vi "InitWrist V2.vi"() -> ()   [LabVIEW 2015]
uses:
  <vilib>/myRIO/Common/Instrument Driver Framework/myRIO v1.0/Encoder/typedefs/Encoder Signal Mode.ctl
  <vilib>/myRIO/Instrument Drivers/Onboard IO/Encoder/typedefs/Encoder Reference.ctl
  <vilib>/myRIO/Common/Instrument Driver Framework/Utilities/typedefs/myRIO Generic Hardware Reference.ctl
  <vilib>/myRIO/Common/Instrument Driver Framework/Utilities/typedefs/Hardware Version Enum.ctl
  <vilib>/myRIO/Common/Instrument Driver Framework/Utilities/typedefs/myRIO v1.0 Reference.ctl
  <vilib>/myRIO/Common/Instrument Driver Framework/Utilities/typedefs/Generic FPGA Reference.ctl
  <vilib>/myRIO/Common/Instrument Driver Framework/myRIO v1.0/Encoder/typedefs/Encoder Channels Enum.ctl
  <vilib>/myRIO/Common/Instrument Driver Framework/myRIO v1.0/Encoder/typedefs/Encoder Configuration v1.0.ctl
  <vilib>/userdefined/High Color/nirio_resource_hc.ctl
  <vilib>/myRIO/Instrument Drivers/Onboard IO/DIO/typedefs/DIO Reference.ctl
  <vilib>/myRIO/Common/Instrument Driver Framework/myRIO v1.0/DIO/typedefs/DIO Channels List.ctl
  <vilib>/myRIO/Common/Instrument Driver Framework/myRIO v1.0/DIO/typedefs/DIO Channels Enum.ctl
  <vilib>/myRIO/Common/Instrument Driver Framework/Utilities/vis/Is FPGA Ref Available.vi
  <vilib>/myRIO/Common/Instrument Driver Framework/myRIO v1.0/Encoder/vis/myRIO v1.1 Open Encoder.vi
  <vilib>/myRIO/Instrument Drivers/Onboard IO/Encoder/vis/Read.vi
  <vilib>/myRIO/Common/Instrument Driver Framework/myRIO v1.0/DIO/vis/myRIO v1.1 Open DIO.vi
  <vilib>/myRIO/Instrument Drivers/Onboard IO/DIO/vis/Read.vi
  <vilib>/myRIO/Common/Instrument Driver Framework/Utilities/vis/Validate Channels.vi
  <vilib>/myRIO/Common/Instrument Driver Framework/myRIO v1.0/Encoder/vis/myRIO v1.0 Reserve Encoder.vi
  <vilib>/myRIO/Common/Instrument Driver Framework/myRIO v1.0/DIO/vis/myRIO v1.0 Reserve DIO.vi
  <vilib>/myRIO/Common/Instrument Driver Framework/myRIO v1.0/Encoder/vis/myRIO v1.0 Build MUX Configuration Encoder.vi
  <vilib>/myRIO/Common/Instrument Driver Framework/myRIO v1.0/Resource Manager/vis/myRIO v1.0 Reserve Channel List.vi
  <vilib>/myRIO/Common/Instrument Driver Framework/myRIO v1.0/DIO/vis/myRIO v1.0 Build MUX Configuration DIO.vi
  <vilib>/myRIO/Common/Instrument Driver Framework/myRIO v1.0/Resource Manager/vis/myRIO v1.0 Create Configuration List.vi
  <vilib>/myRIO/Common/Instrument Driver Framework/myRIO v1.0/Resource Manager/vis/myRIO v1.0 Reserve Channel.vi
  <vilib>/myRIO/Common/Instrument Driver Framework/myRIO v1.0/Resource Manager/vis/myRIO v1.0 Unreserve Channel.vi
  <vilib>/myRIO/Common/Instrument Driver Framework/myRIO v1.0/Resource Manager/vis/myRIO v1.0 Build Mutex Name.vi
  Global Angle.vi
  <vilib>/Utility/VariantDataType/GetNumericInfo.vi
  <vilib>/Utility/error.llb/Error Cluster From Error Code.vi
  <vilib>/myRIO/Common/Instrument Driver Framework/myRIO v1.0/myRIO v1.1 Open.vi
  <vilib>/myRIO/Common/Instrument Driver Framework/Utilities/vis/IO Manager.vi
  <vilib>/myRIO/Common/Instrument Driver Framework/Utilities/vis/Configuration Manager.vi
  <vilib>/myRIO/Common/Instrument Driver Framework/myRIO v1.0/Resource Manager/vis/myRIO v1.0 Configure IO.vi
  <vilib>/myRIO/Common/Instrument Driver Framework/myRIO v1.0/myRIO v1.0 Close.vi
  <vilib>/myRIO/Common/Instrument Driver Framework/myRIO v1.0/Encoder/vis/myRIO v1.0 Configure Encoder.vi
  <vilib>/myRIO/Common/Instrument Driver Framework/myRIO v1.0/Encoder/vis/myRIO v1.0 Read Encoder.vi
  <vilib>/myRIO/Common/Instrument Driver Framework/myRIO v1.0/DIO/vis/myRIO v1.0 Read DIO.vi
  <vilib>/myRIO/Express VI/Onboard IO/Encoder/Encoder Express VI.xnode
  <vilib>/myRIO/Instrument Drivers/Onboard IO/Encoder/vis/myRIO Encoder Open.xnode
  <vilib>/myRIO/Common/Instrument Driver Framework/myRIO v1.0/Encoder/typedefs/Encoder Count Direction Enum.ctl
  <vilib>/myRIO/Express VI/Onboard IO/DI/DI Express VI.xnode
  <vilib>/myRIO/Instrument Drivers/Onboard IO/DIO/vis/myRIO DIO Open.xnode
  <vilib>/myRIO/Instrument Drivers/Onboard IO/Encoder/Encoder.lvlib
  <vilib>/myRIO/Instrument Drivers/Onboard IO/DIO/DIO.lvlib
panel:
  out ".not. x?":bool
  in  "integral":dbl
  out "Boolean":bool
  out "lastError":dbl
  in  "stop":bool
  out "Counter Value":i32
  out "input Rotations":dbl
  out "error":i32
  out "motorStop":bool
  out "differential":i32
  out "output":i32
  out "busy":bool
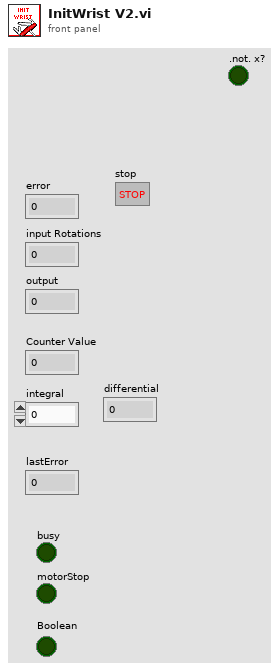
[diagram p1: front panel]
types:
  T1 = typedef "Encoder.lvlib/Encoder Reference.ctl" = cluster{"myRIO Reference":T2, "Encoder Channels Enum":T6}
  T2 = typedef "myRIO Generic Hardware Reference.ctl" = cluster{"myRIO Model":T3, "myRIO Hardware Reference":T4}
  T3 = typedef "Hardware Version Enum.ctl" = enum16{"Unknown", "myRIO-1900", "myRIO-1950", "roboRIO"}
  T4 = typedef "myRIO v1.0 Reference.ctl" = cluster{"Generic FPGA Reference":T5, "Allow multiple opens":bool}
  T5 = typedef "Generic FPGA Reference.ctl" = refnum<k20>
  T6 = typedef "Encoder Channels Enum.ctl" = enum16{"Not Connected", "C/ENC0", "C/ENC1", "A/ENC", "B/ENC", "DIO/ENC0", "DIO/ENC1", "DIO/ENC2", "DIO/ENC3", "DIO/ENC4"}
  T7 = typedef "Encoder Signal Mode.ctl" = enum16{"Quadrature phase signal", "Step and direction signal"}
  T8 = typedef "nirio_resource_hc.ctl" = tag
  T9 = typedef "DIO.lvlib/DIO Reference.ctl" = cluster{"myRIO Reference":T2, "DIO Channels List":T10}
  T10 = typedef "DIO Channels List.ctl" = T11[]
  T11 = typedef "DIO Channels Enum.ctl" = enum16{"Not Connected", "C/DIO0", "C/DIO1", "C/DIO2", "C/DIO3", "C/DIO4", "C/DIO5", "C/DIO6", "C/DIO7", "A/DIO0", "A/DIO1", "A/DIO2", "A/DIO3", "A/DIO4", "A/DIO5", "A/DIO6", "A/DIO7", "A/DIO8", "A/DIO9", "A/DIO10", "A/DIO11", "A/DIO12", "A/DIO13", "A/DIO14", "A/DIO15", "B/DIO0", "B/DIO1", "B/DIO2", "B/DIO3", "B/DIO4", "B/DIO5", "B/DIO6", "B/DIO7", "B/DIO8", "B/DIO9", "B/DIO10", "B/DIO11", "B/DIO12", "B/DIO13", "B/DIO14", "B/DIO15", "LED0", "LED1", "LED2", "LED3", "Button0", "DIO/DIO0", "DIO/DIO1", "DIO/DIO2", "DIO/DIO3", "DIO/DIO4", "DIO/DIO5", "DIO/DIO6", "DIO/DIO7", "DIO/DIO8", "DIO/DIO9", "SPI/CS0", "SPI/CS1", "SPI/CS2", "SPI/CS3", "LED RADIO (Green)", "LED RADIO (Red)", "LED COMM (Green)", "LED COMM (Red)", "LED MODE (Green)", "LED MODE (Red)"}
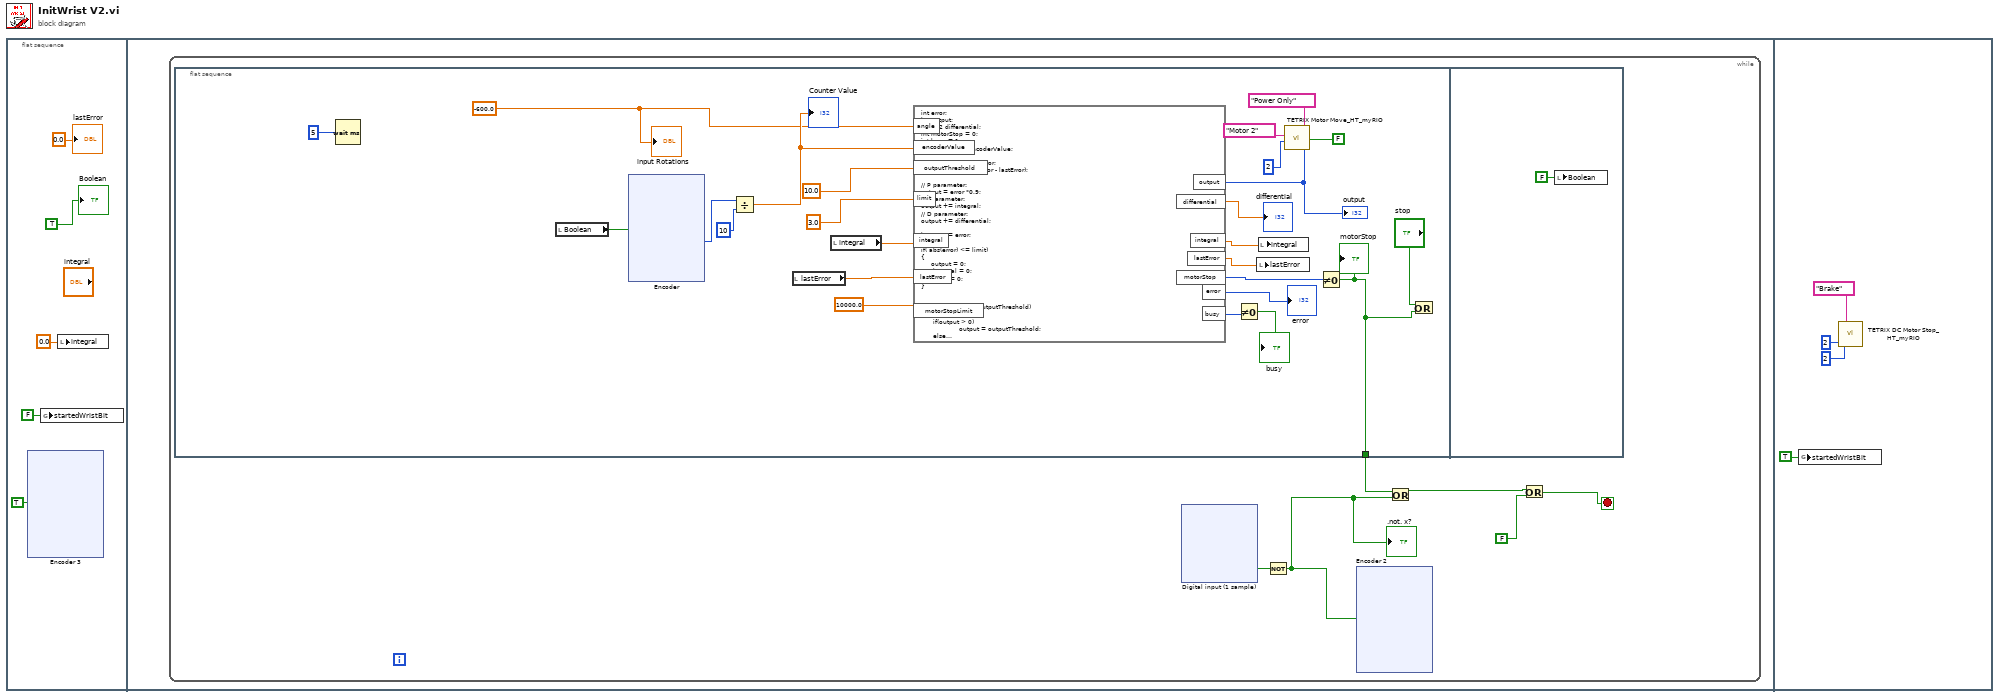
[diagram p0: block diagram]
diagram:
  n1 = flat-sequence {
    frame #0 {
      n2 = xnode "Encoder 3"("Reset Counter"=TRUE) -> ()  [unwired: 1 in, 4 out]
      n3 = global write "Global Angle.vi" "startedWristBit"(FALSE ("startedWristBit")) -> ()
      n4 = local write "integral"(0.0 ("integral")) -> ()
      "lastError" <- 0.0 ("lastError")
      "Boolean" <- TRUE ("Boolean")
    }
    frame #1 {
      n5 = while {
        stop <- w53 stop-if-true
        n6 = flat-sequence {
          tunnel: [w140] -> w57
          frame #0 {
            w145 = -600.0 ("input variable")
            n7 = Wait (ms)(milliseconds to wait=u32 5) -> ()  [unwired: 1 out]
            n8 = local read "Boolean"() -> (w148:bool)
            n9 = xnode "Encoder"("Reset Counter"=w148) -> ("Counter Value"=w157:i32)  [unwired: 1 in, 3 out]
            n10 = Divide(x=w157, y=10) -> (x/y=w155:dbl)
            "Counter Value" <- w155
            n11 = local read "lastError"() -> (w159:dbl)
            n12 = local read "integral"() -> (w142:dbl)
            n13 = formula code="int error;\nint output;\nfloat32 differential;\nint motorStop = 0;\nint busy = 1;\nerror = angle - encoderValue;\n\nintegral += 0.008*error;\ndifferential = 0.6*(error - lastError);\n\n// P parameter:\noutput = error *0.9;\n// I parameter:\noutput += integral;\n// D parameter:\noutput += differential;\n\nlastError = error;\n\nif( abs(error) <= limit)\n{\n     output = 0;\n      integral = 0;\n      busy = 0;\n}\n \n\nif( abs(output) >= outputThreshold)\n {\n      if(output > 0)\n                   output = outputThreshold;\n      else \n                  output = -1*outputThreshold;\n}\n\nif(abs(integral) >= motorStopLimit && abs(differential)  <= 0.06)\n      motorStop = 1;"("angle"=w145, "encoderValue"=w155, "outputThreshold"=10.0 ("input variable"), "limit"=3.0 ("input variable"), "integral"=w142, "lastError"=w159, "motorStopLimit"=10000.0 ("input variable")) -> ("output"=w141:i32, "integral"=w144:dbl, "lastError"=w143:dbl, "error"=→"error":i32, "motorStop"=w153:i32, "differential"=→"differential":sgl, "busy"=w147:i32)
            "output" <- w141
            n14 = Not Equal To 0?(x=w147) -> (x != 0?=→"busy":bool)
            n15 = local write "lastError"(w143) -> ()
            n16 = local write "integral"(w144) -> ()
            n17 = call <vilib>:"TETRIX Motor Move_HT_myRIO.vi"("Power (-100 to 100)\n0 = Stop/Brake\n-128 = Stop/Coast"=w141, "Reverse? : T or F"=FALSE, "Control Mode"="Power Only", "Controller Daisy Chain Position: 1 - 4"=u8 2, "Select Channel"="Motor 2") -> ()  [unwired: 2 in, 1 out]
            n18 = Not Equal To 0?(x=w153) -> (x != 0?=w140:bool)
            "motorStop" <- w140
            n19 = Or(x="stop", y=w140) -> ()  [unwired: 1 out]
            "input Rotations" <- w145
          }
          frame #1 {
            n20 = local write "Boolean"(FALSE ("Boolean")) -> ()
          }
        }
        n21 = xnode "Digital input (1 sample)"() -> ("A/DIO1 (Pin 13)"=w56:bool)  [unwired: 1 in, 1 out]
        n22 = Not(x=w56) -> (.not. x?=w55:bool)
        ".not. x?" <- w55
        n23 = xnode "Encoder 2"("Reset Counter"=w55) -> ()  [unwired: 1 in, 4 out]
        n24 = Or(x=w57, y=w55) -> (x .or. y?=w54:bool)
        n25 = Or(x=w54, y=FALSE) -> (x .or. y?=w53:bool)
      }
    }
    frame #2 {
      n26 = global write "Global Angle.vi" "startedWristBit"(TRUE ("startedWristBit")) -> ()
      n27 = call <vilib>:"TETRIX DC Motor Stop_HT_myRIO.vi"("Stop (Brake or Coast)"="Brake", "Motor Channel: (1 or 2)"=u8 2, "Controller Daisy Chain Position: 1 - 4"=u8 2) -> ()  [unwired: 1 in, 1 out]
    }
  }
